vi "Rec_set dialog.vi"(8 "错误输入（无错误）":errorcluster) -> (0 "错误输出":errorcluster, 2 "参数设置 out":T1={"测量模式"=enum."force clamp", "测量起点"=0.0, "数据存放路径"=path "", "加载率(pN/s)"=0.01, "初始转数"=0.0, "最终转数"=0.0, "旋转速度"=0.0, "步长"=0.0, "FC停留时间"=0.0, "实验名称"="", "往返？"=FALSE, "驰豫时间（s）"=0.0, "单位"=enum."分", "测量周期"=0, "驰豫位置"=0.0, "FR每步时间(s)"=0.5, "测量终点"=[], "阶段终点"=[1.4, 1.0, 0.7], "阶段等待时间(s)"=[3.0, 2.0, 1.0], "顶端驰豫时间"=0, "顶端驰豫"=FALSE} {"FR每步时间(s)" min=0.5; "加载率(pN/s)" min=0.01}, 3 "Cancelled?":bool caption="取消？")   [LabVIEW 2017]
doc: "该模板用于创建能够进行事件处理的对话框。"
uses:
  control/record mode.ctl
  parameter set for record.ctl
panel:
  in  "顶端驰豫时间(s)":u32=60
  in  "顶端驰豫":bool
  in  "阶段等待时间(s)":dbl[](array[numeric])
  in  "阶段终点":dbl[](array[numeric])
  in  "测量终点":dbl[](array[numeric])
  in  "每步时间(s)":dbl=1.5 min=0.5
  in  "测量模式":T2=enum."force-mixed"
  in  "停留时间单位":enum16{"秒", "毫秒", "分"}(ring)
  in  "往返？":bool
  in  "驰豫位置":dbl=6.0
  in  "驰豫时间（s）":dbl=200.0
  in  "测量周期":i32=3
  in  "实验名称":string
  in  "Cancel":bool caption="取消"
  in  "OK":bool caption="确定"
  in  "步长":dbl=-0.005
  in  "数据存放路径":path=path "D:/辅助软件/test data"
  in  "测量起点":dbl=4.0
  in  "加载率":dbl=0.1
  in  "停留时间":dbl=2.0
  # "通用"
  # "force ramp"
  # "force time set"
  # "force clamp"
  # "force ramp"
  # "force ramp"
  # "通用"
  # "force ramp"
  # "force clamp"
  # "磁铁旋转"
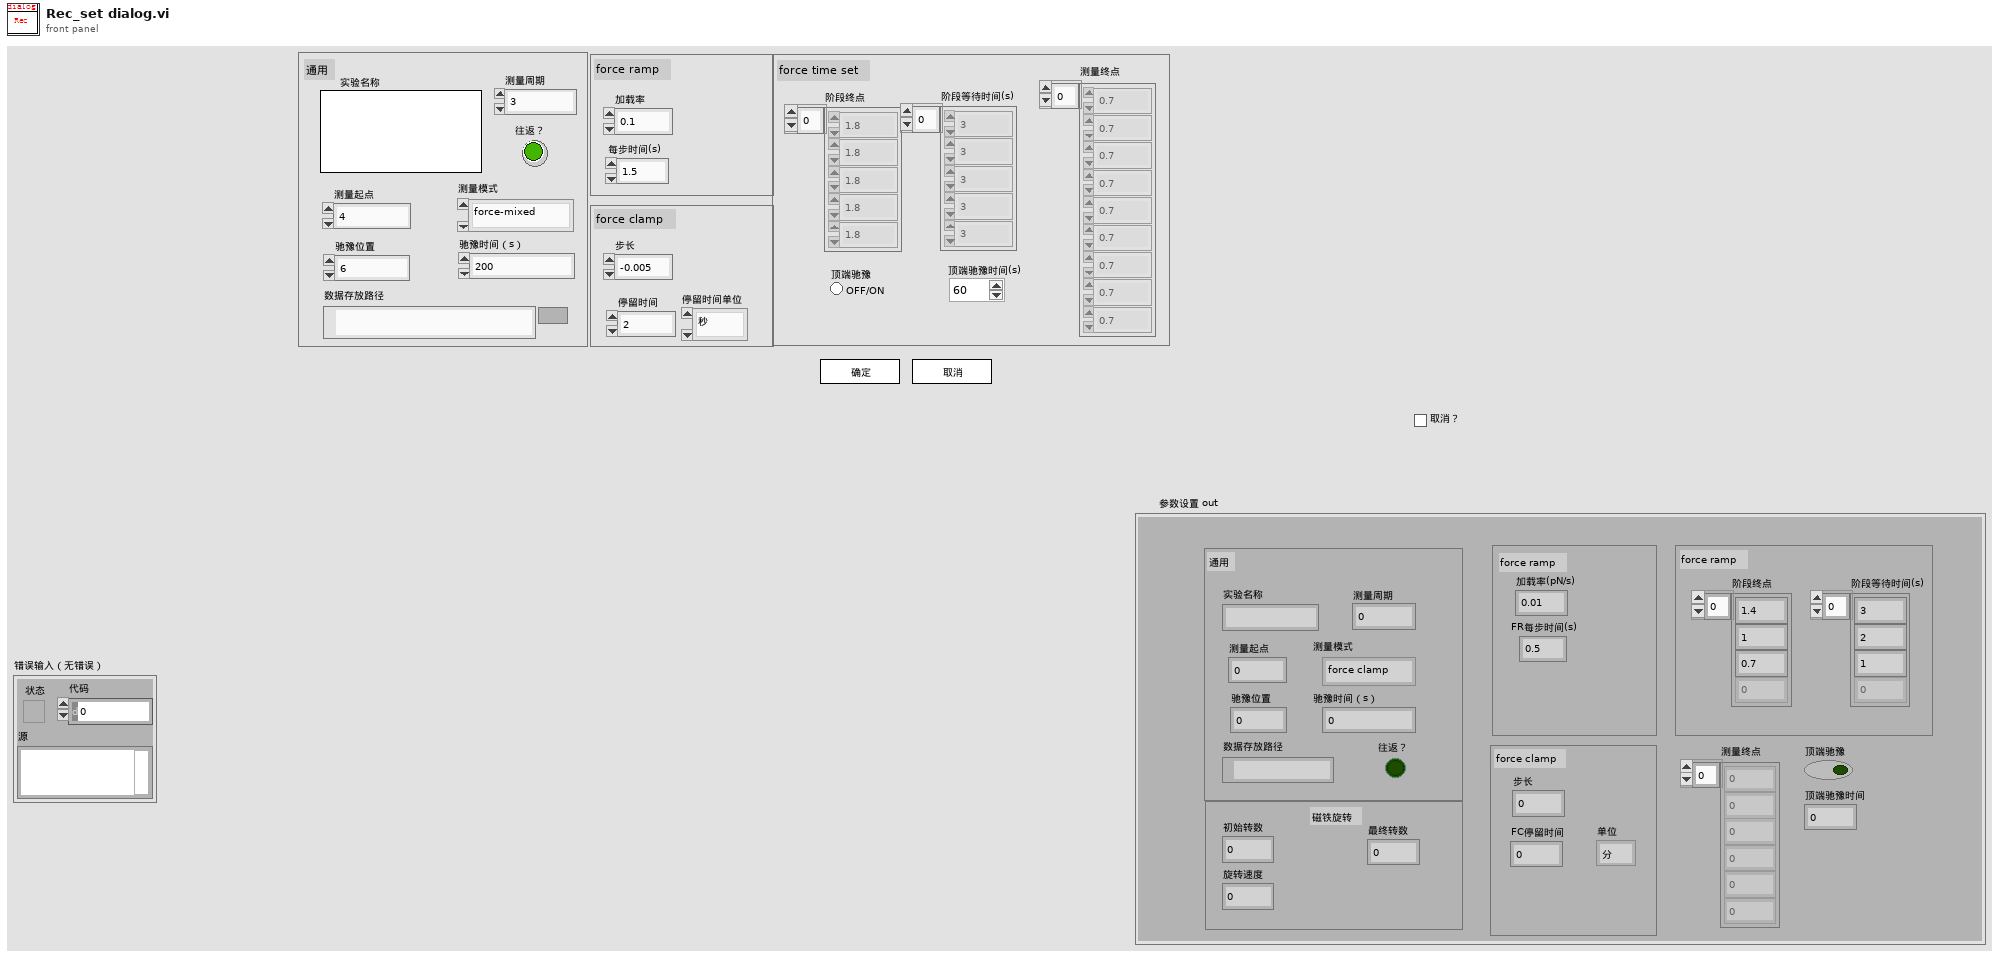
[diagram p1: front panel]
types:
  T1 = typedef "parameter set for record.ctl" = cluster{"测量模式":T2, "测量起点":dbl, "数据存放路径":path, "加载率(pN/s)":dbl, "初始转数":dbl, "最终转数":dbl, "旋转速度":dbl, "步长":dbl, "FC停留时间":dbl, "实验名称":string, "往返？":bool, "驰豫时间（s）":dbl, "单位":enum16{"秒", "毫秒", "分"}, "测量周期":i32, "驰豫位置":dbl, "FR每步时间(s)":dbl, "测量终点":dbl[], "阶段终点":dbl[], "阶段等待时间(s)":dbl[], "顶端驰豫时间":u32, "顶端驰豫":bool}
  T2 = typedef "record mode.ctl" = enum16{"force ramp", "force clamp", "user-defined", "force-mixed"}
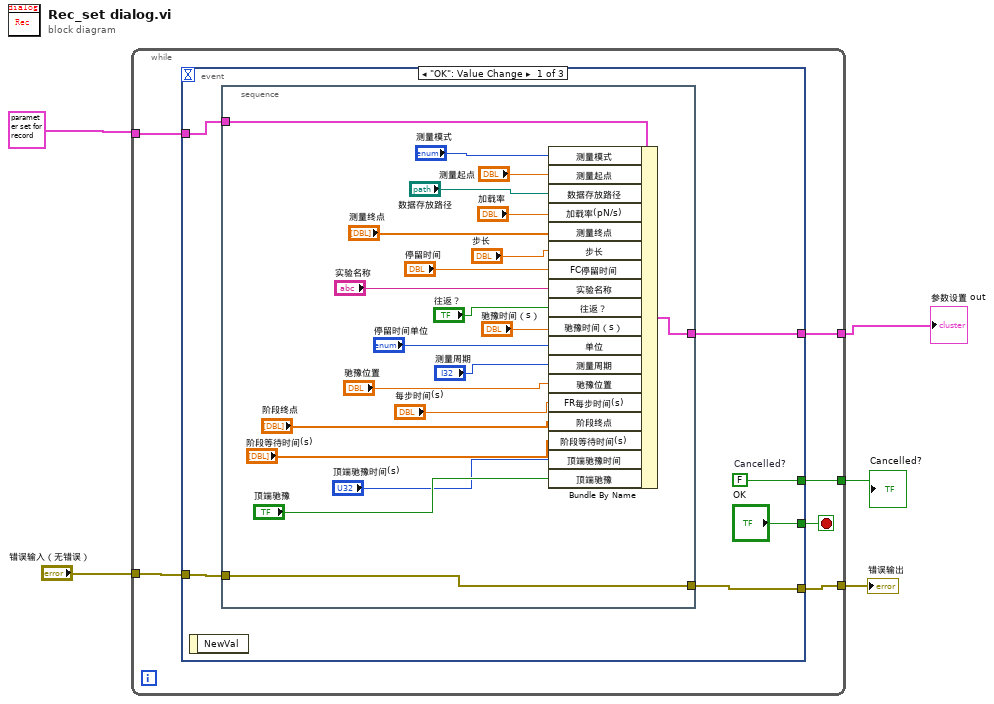
[diagram p0: block diagram]
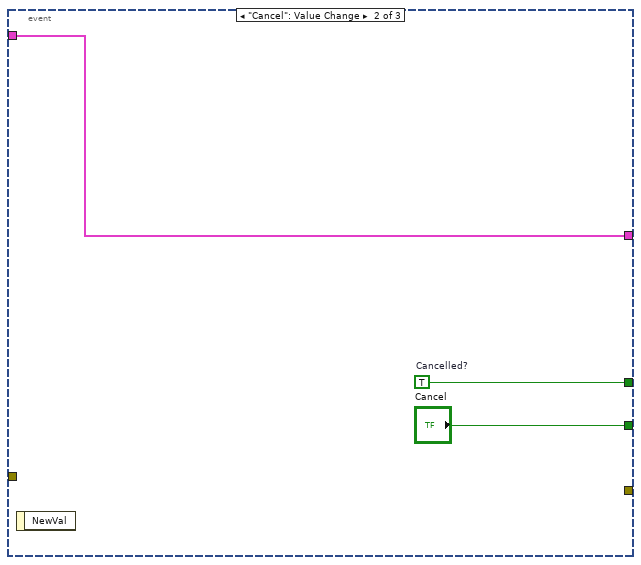
[diagram p2: hidden frame]
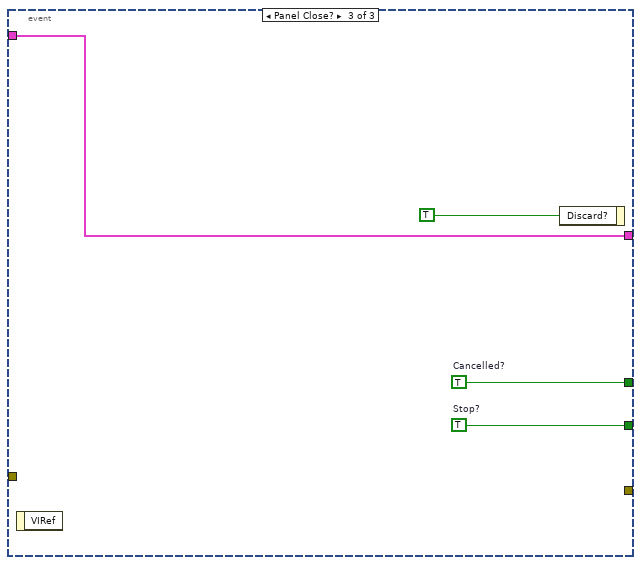
[diagram p3: hidden frame]
diagram:
  n1 = while {
    tunnel: [w10] -> w5
    tunnel: [w9] -> w1
    tunnel: T1 {"测量模式"=enum."force clamp", "测量起点"=0.0, "数据存放路径"=path "", "加载率(pN/s)"=0.01, "初始转数"=0.0, "最终转数"=0.0, "旋转速度"=0.0, "步长"=0.0, "FC停留时间"=0.0, "实验名称"="", "往返？"=FALSE, "驰豫时间（s）"=0.0, "单位"=enum."分", "测量周期"=0, "驰豫位置"=0.0, "FR每步时间(s)"=0.5, "测量终点"=[], "阶段终点"=[1.4, 1.0, 0.7], "阶段等待时间(s)"=[3.0, 2.0, 1.0], "顶端驰豫时间"=0, "顶端驰豫"=FALSE} ("参数设置 in") -> [w8]
    tunnel: "错误输入（无错误）" -> [w7]
    tunnel: [w6] -> w3
    stop <- w11 stop-if-true
    n2 = event shown="[0] \"OK\": Value Change" {
      selector: _ -> [_ _ _]
      dyn-events: _ -> [_ _ _]
      timeout: _ -> [_ _ _]
      tunnel: ["OK" "Cancel" w44] -> w11
      tunnel: [w17 w41 w43] -> w10
      tunnel: [w14 w39 w42] -> w9
      tunnel: w8 -> [w15 w39 w42]
      tunnel: w7 -> [w13 _ _]
      tunnel: [w12 _ _] -> w6
      event "OK": Value Change {
        w17 = FALSE  # Cancelled?
        n3 = event-data() -> ()  [unwired: 1 in, 1 out]
        n4 = stacked-sequence {
          tunnel: [w38] -> w14
          tunnel: w15 -> [w33]
          tunnel: w13 -> [w32]
          tunnel: [w32] -> w12
          frame #0 {
            n5 = Bundle By Name(cluster=w33, "测量模式"="测量模式", "测量起点"="测量起点", "数据存放路径"="数据存放路径", "加载率(pN/s)"="加载率", "测量终点"="测量终点", "步长"="步长", "FC停留时间"="停留时间", "实验名称"="实验名称", "往返？"="往返？", "驰豫时间（s）"="驰豫时间（s）", "单位"="停留时间单位", "测量周期"="测量周期", "驰豫位置"="驰豫位置", "FR每步时间(s)"="每步时间(s)", "阶段终点"="阶段终点", "阶段等待时间(s)"="阶段等待时间(s)", "顶端驰豫时间"="顶端驰豫时间(s)", "顶端驰豫"="顶端驰豫") -> (w38:T1)
          }
        }
      }
      event "Cancel": Value Change {
        w41 = TRUE  # Cancelled?
        n6 = event-data() -> ()  [unwired: 1 in, 1 out]
      }
      event Panel Close? {
        w43 = TRUE  # Cancelled?
        w44 = TRUE  # Stop?
        n7 = event-data() -> ()  [unwired: 1 in, 1 out]
        n8 = event-data("Discard?"=TRUE) -> ()  [unwired: 1 in, 1 out]
      }
    }
  }
  "Cancelled?" <- w5
  "错误输出" <- w3
  "参数设置 out" <- w1
